vi "Test Discard Old Elements on Overflow.vi"(8 "error in (no error)":errorcluster, 11 "Test Case In":refnum<class "Debug Log Test.lvclass">) -> (0 "error out":errorcluster, 3 "Test Case Out":refnum<class "Debug Log Test.lvclass">)   [LabVIEW 2020, in "Debug Log Test.lvclass"]
uses:
  Debug Log Test.lvclass
  C:/Program Files (x86)/National Instruments/LabVIEW 2020/vi.lib/Astemes/LUnit/Test Case.lvclass
  source/Debug Log/Debug Log.lvclass
  source/Debug Log/Debug Log.lvclass/Debug Log.ctl
  source/Debug Data/Debug Data.lvclass/Debug Data.ctl
  <vilib>/Astemes/LUnit/Test Case.lvclass/Test Case.ctl
  <vilib>/Astemes/LUnit/LUnit Assertion Result.lvclass/LUnit Assertion Result.ctl
  <vilib>/Astemes/LUnit/LUnit Test Case Result.lvclass/LUnit Test Case Result.ctl
  <vilib>/Astemes/LUnit/LUnit Method Result.lvclass/LUnit Method Result.ctl
  01074fa8-ee8a-411d-bc8b-fc92c4f90959.vi
  e110ba72-c4f9-4de7-bf05-3ebd5ee4e4e5.vi
  source/Debug Log/Read Unfiltered Log Content.vi
  <vilib>/Astemes/LUnit/Palette/Pass.vi
  <vilib>/Astemes/LUnit/Palette/Fail.vi
  <vilib>/Astemes/LUnit/Compare Variants.vi
  <vilib>/Astemes/LUnit/Describe Comparison.vi
  <vilib>/Astemes/LUnit/Set Assertion Type.vi
  <vilib>/Astemes/LUnit/Add test result.vi
  <vilib>/Astemes/LUnit/LUnit Write Passed.vi
  <vilib>/Astemes/LUnit/LUnit Write Message.vi
  <vilib>/Astemes/LUnit/LUnit Write Description.vi
  <vilib>/Astemes/LUnit/Variant to string.vi
  <vilib>/Astemes/LUnit/LUnit Write Assertion Type.vi
  <vilib>/Astemes/LUnit/LUnit Record Assertion Result.vi
  <vilib>/Astemes/LUnit/LUnit Aggregate Assertion Results.vi
  <vilib>/Astemes/LUnit/Assertion Result/LUnit Read Status.vi
  <vilib>/Astemes/LUnit/LUnit Read Message.vi
  <vilib>/Astemes/LUnit/LUnit Read Description.vi
  <vilib>/Astemes/LUnit/Method Result/LUnit Merge Status.vi
  <vilib>/Astemes/LUnit/LUnit Concatenate result strings.vi
  <vilib>/Utility/Data Type/Get Type Information.vi
  <vilib>/Utility/LVClass/Get LV Class Name.vi
  <vilib>/Astemes/LUnit/LUnit Assertion Result.lvclass
  source/Filter/Filter.lvclass
  source/Debug Data/Debug Data.lvclass
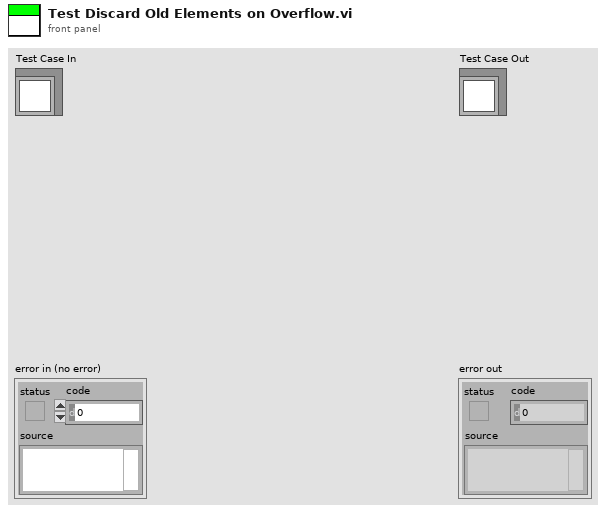
[diagram p1: front panel]
types:
  T1 = cluster{"Action":string, "Call Chain":string, "Process":string, "Message":string, "Message Data":variant, "Time":u32}[]
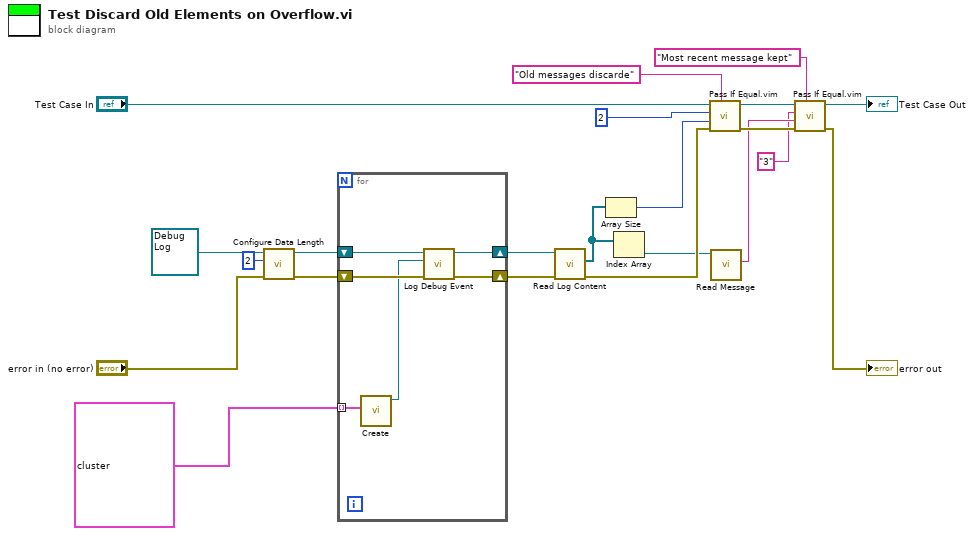
[diagram p0: block diagram]
diagram:
  n1 = call "Configure Data Length.vi"("error in (no error)"="error in (no error)", "Data Length"=2, "Debug Log In"=refnum<class "Debug Log.lvclass"> refnum ("Debug Log.lvclass")) -> ("error out"=w15:errorcluster, "Debug Log Out"=w17:refnum<class "Debug Log.lvclass">)  [unwired: 7 in]
  n2 = for {
    tunnel: T1 [{"Action"="", "Call Chain"="", "Process"="", "Message"="1", "Message Data"=variant, "Time"=0}, {"Action"="", "Call Chain"="", "Process"="", "Message"="2", "Message Data"=variant, "Time"=0}, {"Action"="", "Call Chain"="", "Process"="", "Message"="3", "Message Data"=variant, "Time"=0}] ("Debug Data Cluster") -> [w24] mode=indexing
    shift-right: [w27] -> w16
    shift-left: w17 -> [w28]
    shift-right: [w25] -> w14
    shift-left: w15 -> [w26]
    n3 = call "Create.vi"("Debug Data Cluster"=w24) -> ("Debug Data out"=w23:refnum<class "Debug Data.lvclass">)  [unwired: 9 in, 1 out]
    n4 = call "Log Debug Event.vi"("error in (no error)"=w26, "Debug Data.lvclass"=w23, "Debugger in"=w28) -> ("error out"=w25:errorcluster, "Debugger out"=w27:refnum<class "Debug Log.lvclass">)  [unwired: 7 in]
  }
  n5 = call "Read Log Content.vi"("error in (no error)"=w14, "Debug Log In"=w16) -> ("error out"=w18:errorcluster, "Data Log"=w6:refnum<class "Debug Data.lvclass">[])  [unwired: 7 in, 1 out]
  n6 = Array Size(array=w6) -> (size(s)=w12:i32)
  n7 = Index Array(array=w6) -> (element=w5:refnum<class "Debug Data.lvclass">)  [unwired: 1 in]
  n8 = call "Pass If Equal.vim"("Description"="Old messages discarde", "error in (no error)"=w18, "Actual"=w12, "Expected"=2 ("size(s)"), "LUnit Test Case In"="Test Case In") -> ("error out"=w8:errorcluster, "LUnit Test Case Out"=w10:refnum<class "Debug Log Test.lvclass">)  [unwired: 5 in]
  n9 = call "Read Message.vi"("Debug Data in"=w5) -> ("Message"=w4:string)  [unwired: 8 in, 2 out]
  n10 = call "Pass If Equal.vim"("Description"="Most recent message kept", "error in (no error)"=w8, "Actual"=w4, "Expected"="3", "LUnit Test Case In"=w10) -> ("error out"=→"error out":errorcluster, "LUnit Test Case Out"=→"Test Case Out":refnum<class "Debug Log Test.lvclass">)  [unwired: 5 in]
